vi "convert_polar_to_rectangular.vi"(3 "error in":errorcluster, 4 "Laser Packet":T1) -> (0 "error out":errorcluster, 1 "Cartesian Coordinates":cluster{"X":sgl, "Y":sgl, "Z":sgl})   [LabVIEW 2019]
doc: "Converts polar coordinates from the Velodyne to rectagular."
panel:
  in  "3D Point":cluster{"X":sgl, "Y":sgl, "Z":sgl}
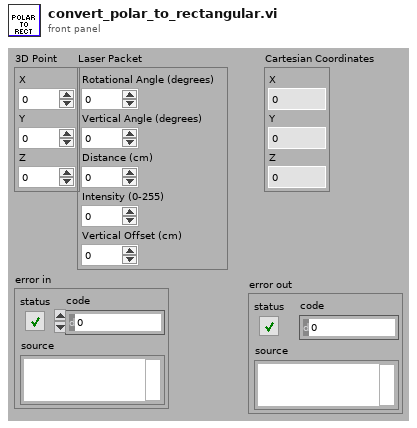
[diagram p1: front panel]
types:
  T1 = cluster{"Rotational Angle (degrees)":dbl, "Vertical Angle (degrees)":dbl, "Distance (cm)":dbl, "Intensity (0-255)":u8, "Vertical Offset (cm)":dbl}
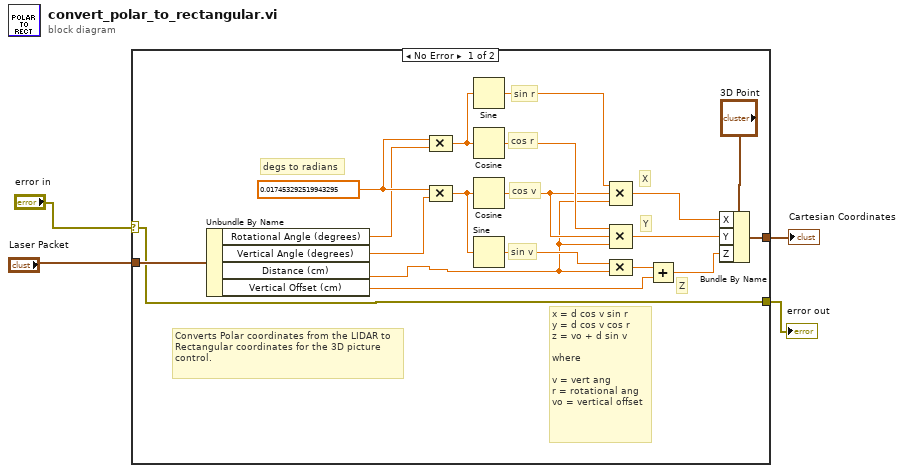
[diagram p0: block diagram]
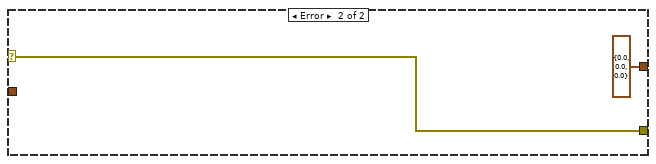
[diagram p2: hidden frame]
diagram:
  n1 = case shown="No Error" "error in" {
    selector: "error in" -> [w6 w24]
    tunnel: [w11 cluster{"X":sgl, "Y":sgl, "Z":sgl} {"X"=0.0, "Y"=0.0, "Z"=0.0} ("3D Point")] -> w4
    tunnel: "Laser Packet" -> [w7 _]
    tunnel: [w6 w24] -> w1
    frame No Error {
      w14 = 0.017453292519943295 ("x/y")
      # "Converts Polar coordinates from the LIDAR to Rectangular coordinates for the 3D picture control."
      # "sin v"
      # "cos v"
      # "cos r"
      # "sin r"
      # "Z"
      # "Y"
      # "X"
      # "degs to radians"
      # "x = d cos v sin r\ny = d cos v cos r\nz = vo + d sin v\n\nwhere\n\nv = vert ang\nr = rotational ang\nvo = vertical offset"
      n2 = Unbundle By Name(w7) -> ("Rotational Angle (degrees)"=w13:dbl, "Vertical Angle (degrees)"=w15:dbl, "Distance (cm)"=w5:dbl, "Vertical Offset (cm)"=w8:dbl)
      n3 = Compound Arithmetic op=MULTIPLY(w14, w13) -> (w17:dbl)
      n4 = Compound Arithmetic op=MULTIPLY(w14, w15) -> (w16:dbl)
      n5 = Sine(x=w17) -> (sin(x)=w18:dbl)
      n6 = Cosine(x=w17) -> (cos(x)=w20:dbl)
      n7 = Cosine(x=w16) -> (cos(x)=w19:dbl)
      n8 = Sine(x=w16) -> (sin(x)=w21:dbl)
      n9 = Compound Arithmetic op=MULTIPLY(w18, w19, w5) -> (w22:dbl)
      n10 = Compound Arithmetic op=MULTIPLY(w20, w19, w5) -> (w23:dbl)
      n11 = Compound Arithmetic op=MULTIPLY(w21, w5) -> (w10:dbl)
      n12 = Add(x=w10, y=w8) -> (x+y=w9:dbl)
      n13 = Bundle By Name(cluster="3D Point", "X"=w22, "Y"=w23, "Z"=w9) -> (w11:cluster{"X":sgl, "Y":sgl, "Z":sgl})
    }
    frame Error {
    }
  }
  "Cartesian Coordinates" <- w4
  "error out" <- w1
